vi "声音采集程序.vi"() -> ()   [LabVIEW 2012]
uses:
  <vilib>/sound2/lvsound2.llb/Sampling Mode.ctl
  <vilib>/sound2/lvsound2.llb/Sound Data Format.ctl
  <vilib>/sound2/lvsound2.llb/Sound File Read (DBL).vi
  <vilib>/sound2/lvsound2.llb/Sound File Read Open.vi
  <vilib>/sound2/lvsound2.llb/Sound Output Set Volume (Single).vi
  <vilib>/sound2/lvsound2.llb/Sound Output Write (DBL).vi
panel:
  in  "path":path=path "C:/Users/Administrator/Desktop/声音/support/sample.wav" caption="路径"
  in  "停止 3":bool
  in  "音量 2":dbl(slide)=50.0 scale=0.0..100.0
  in  "设备ID 2":u32
  out "波形图":waveform(dbl)[](graph)
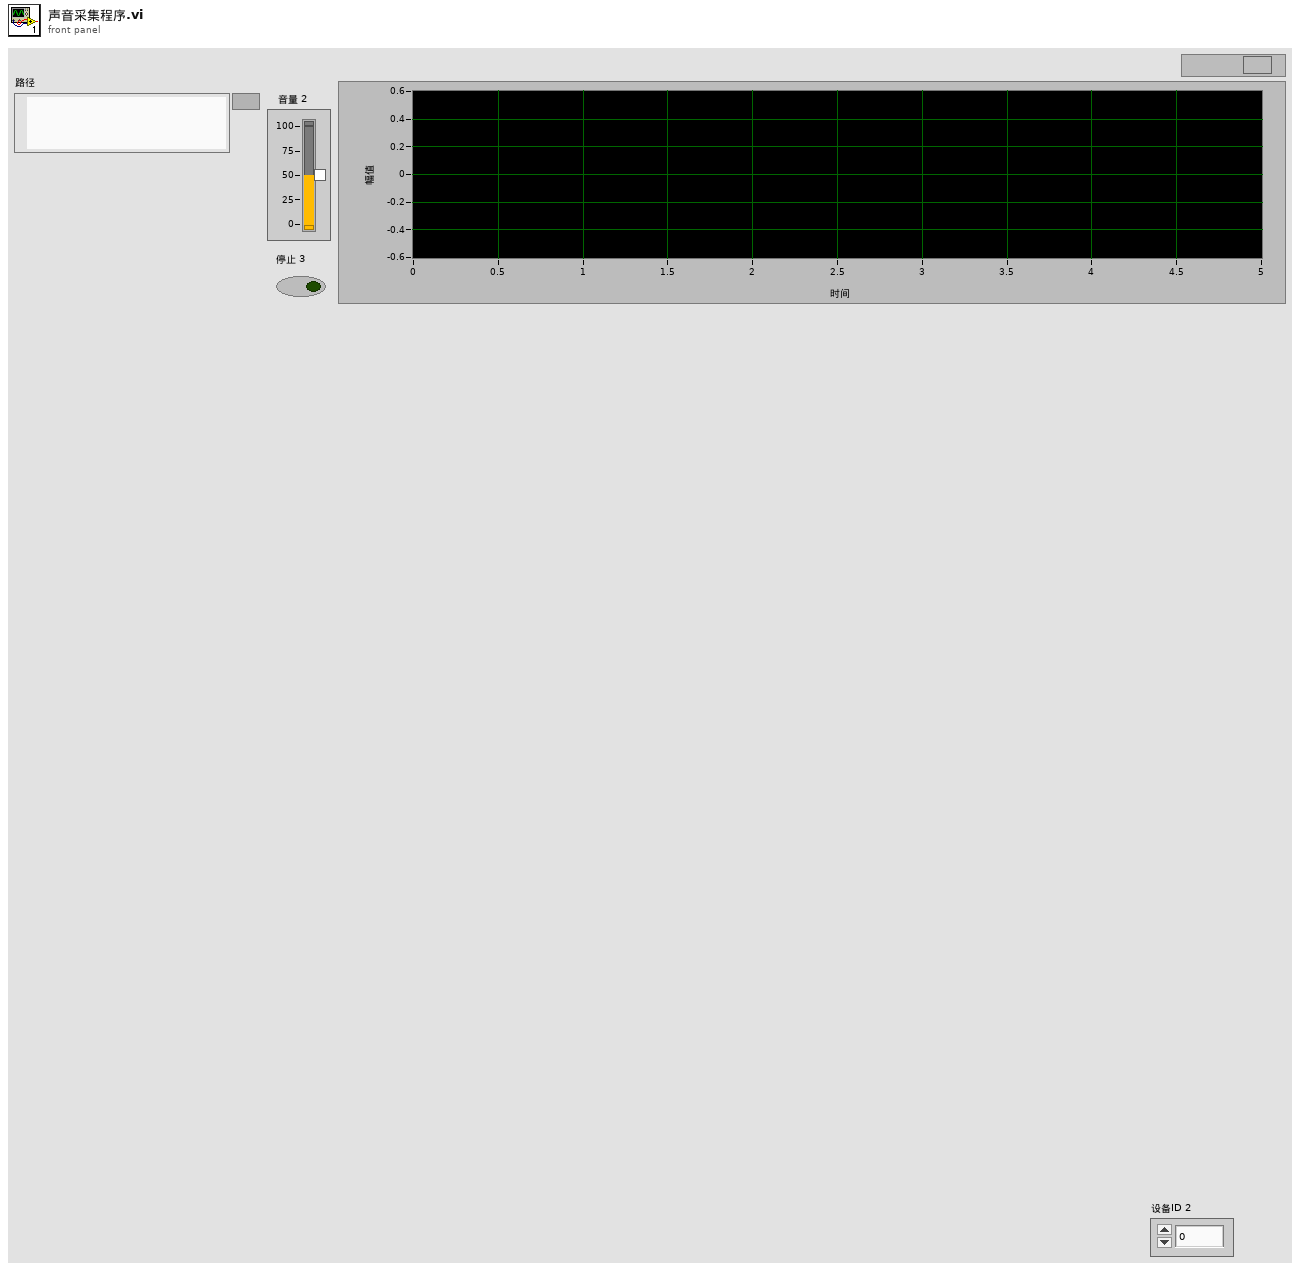
[diagram p1: front panel]
types:
  T1 = typedef "Sound Data Format.ctl" = cluster{"sample rate (S/s)":dbl, "number of channels":i32, "bits per sample":i32}
  T2 = typedef "Sampling Mode.ctl" = i32
  T3 = typedef "Sound Output Task ID.ctl" = u32
  T4 = typedef "Sound File Refnum.ctl" = refnum<file>
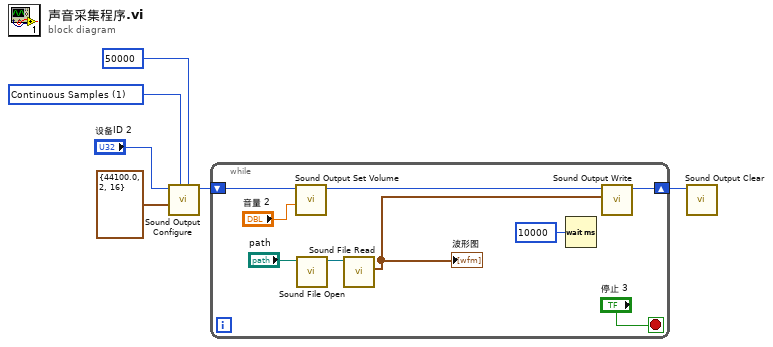
[diagram p0: block diagram]
diagram:
  w2 = T2 1 items=["Finite Samples", "Continuous Samples"] ("sample mode")
  n1 = call <vilib>:"Sound Output Configure.vi"("number of samples/ch"=50000 ("Number of Samples/ch"), "sample mode"=w2, "sound format"=T1 {"sample rate (S/s)"=44100.0, "number of channels"=2, "bits per sample"=16} ("Sound Format"), "device ID"="设备ID 2") -> ("task ID"=w5:T3)  [unwired: 6 in, 1 out]
  n2 = while {
    shift-right: [w9] -> w6
    shift-left: w5 -> [w10]
    stop <- "停止 3" stop-if-true
    n3 = call-poly <vilib>:"Sound Output Set Volume.vi"("volume"="音量 2", "task ID"=w10) -> ("task ID out"=w11:T3)  [unwired: 8 in, 1 out]
    n4 = call-poly <vilib>:"Sound File Open.vi"("path"="path") -> ("sound file refnum"=w14:T4)  [unwired: 9 in, 1 out]
    n5 = call-poly <vilib>:"Sound File Read.vi"("sound file refnum"=w14) -> ("data"=w8:waveform(dbl)[])  [unwired: 6 in, 4 out]
    "波形图" <- w8
    n6 = Wait (ms)(milliseconds to wait=u32 10000 ("等待时间（毫秒）")) -> ()  [unwired: 1 out]
    n7 = call-poly <vilib>:"Sound Output Write.vi"("data"=w8, "task ID"=w11) -> ("task ID out"=w9:T3)  [unwired: 8 in, 1 out]
  }
  n8 = call <vilib>:"Sound Output Clear.vi"("task ID"=w6) -> ()  [unwired: 10 in, 1 out]
